vi "LVClass_CorrectionDataManager GetWavefrontCorrectorCurrentPreferences.vi"(0 "CorrectionDataManager in":refnum<class "CorrectionDataManager.lvclass">, 11 "error in (no error)":errorcluster) -> (4 "CorrectionDataManager out":refnum<class "CorrectionDataManager.lvclass">, 8 "Wavefront Corrector State":T1[](array[typedef]), 15 "error out":errorcluster)   [LabVIEW 2020, in "CorrectionDataManager.lvclass"]
doc: "Wavefront corrector actuators preferences getter.\n\n<B>corrdata_managerIn</B> : CorrDataManager object\n<B>corrdata_managerOut</B> : CorrDataManager object\n<B>min</B> : WavefrontCorrector preferences : lowest command value.\n<B>max</B> : WavefrontCorrector preferences : highest command value.\n<B>validity</B> : WavefrontCorrector preferences : status.\n<B>fixed_value</B> : WavefrontCorrector preferences : fixed positions."
uses:
  CorrectionDataManager.lvclass
  Wavefront Corrector states - ONE.ctl
  CorrectionDataManager.lvclass/CorrectionDataManager.ctl
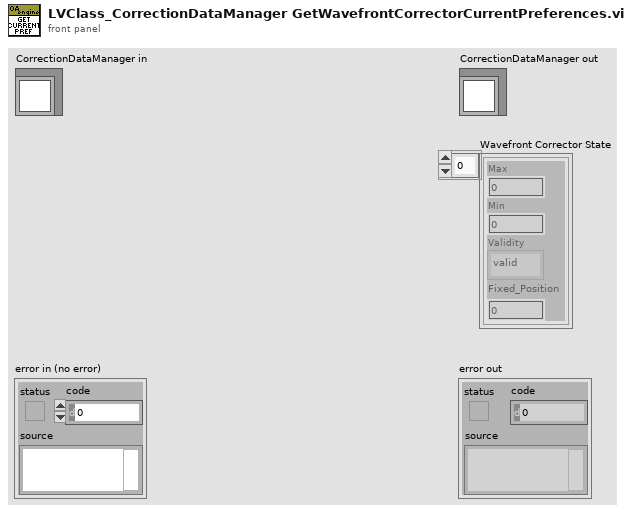
[diagram p1: front panel]
types:
  T1 = typedef "Wavefront Corrector states - ONE.ctl" = cluster{"Max":sgl, "Min":sgl, "Validity":enum16{"valid", "fixed", "invalid"}, "Fixed_Position":sgl}
  T2 = typedef "ClassID.ctl" = i64
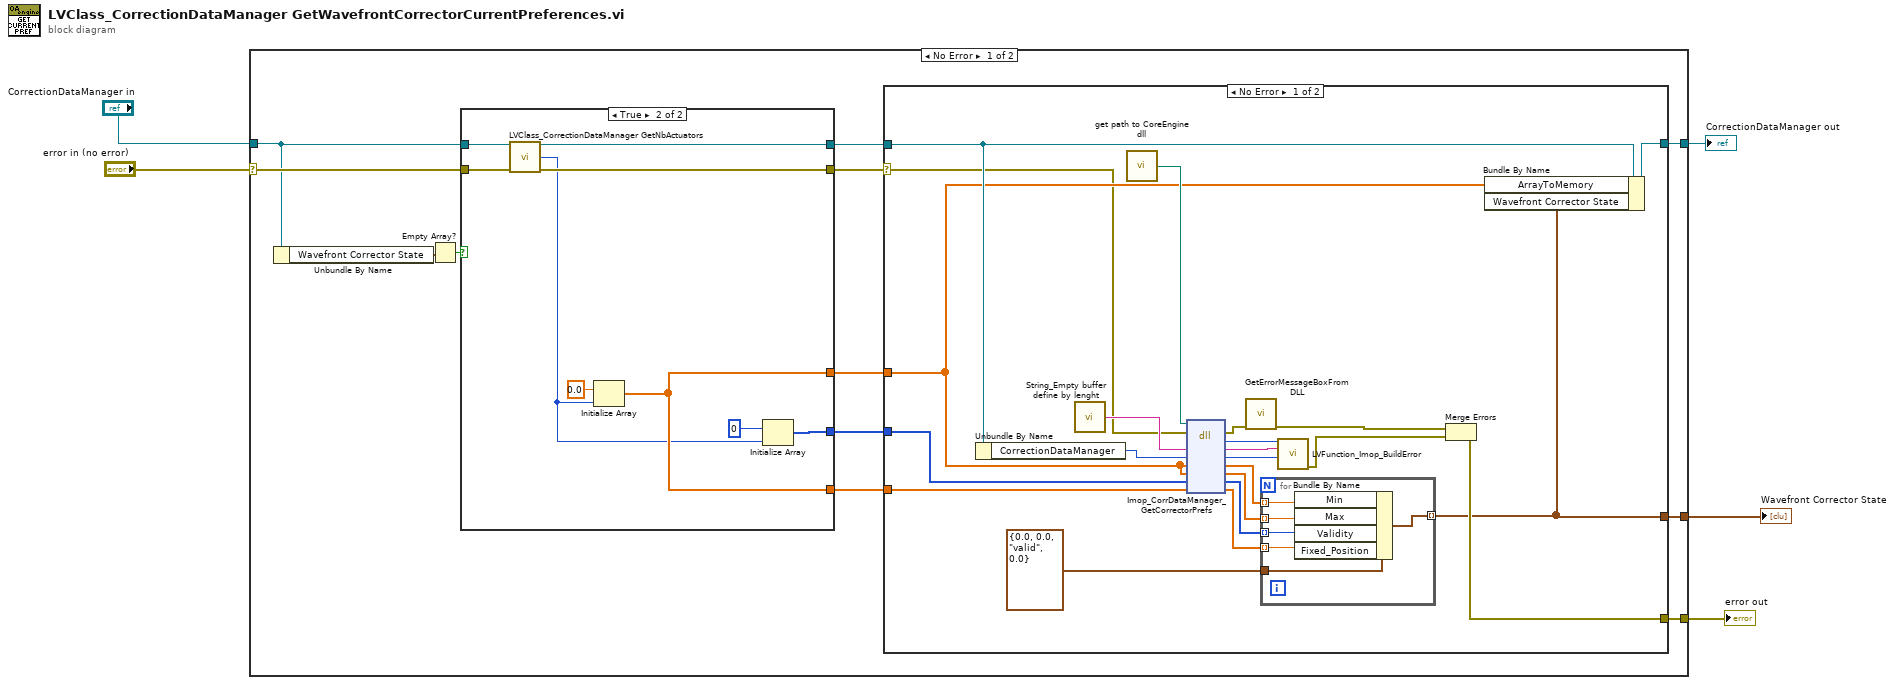
[diagram p0: block diagram]
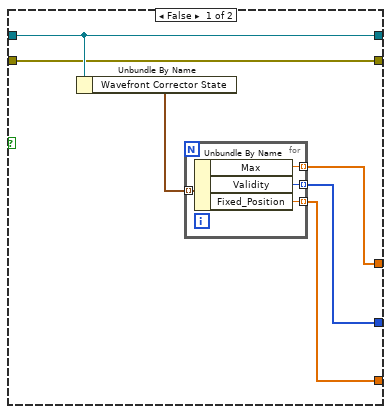
[diagram p3: hidden frame]
diagram:
  n1 = case shown="No Error" "error in (no error)" {
    selector: "error in (no error)" -> [w14 w68]
    tunnel: [w17 w68] -> w4
    tunnel: [w9 w67] -> w5
    tunnel: "CorrectionDataManager in" -> [w13 w67]
    tunnel: [w8 _] -> w1
    frame No Error {
      n2 = Unbundle By Name(w13) -> ("Wavefront Corrector State"=w16:T1[])
      n3 = Empty Array?(array=w16) -> (empty?=w15:bool)
      n4 = case shown="True" w15 {
        tunnel: w13 -> [w53 w64]
        tunnel: [w53 w58] -> w10
        tunnel: [w51 w60] -> w7
        tunnel: [w49 w60] -> w12
        tunnel: w14 -> [w52 w63]
        tunnel: [w52 w62] -> w6
        tunnel: [w50 w61] -> w11
        frame False {
          n5 = Unbundle By Name(w53) -> ("Wavefront Corrector State"=w48:T1[])
          n6 = for {
            tunnel: w48 -> [w57] mode=indexing
            tunnel: [w56] -> w51 mode=indexing
            tunnel: [w55] -> w50 mode=indexing
            tunnel: [w54] -> w49 mode=indexing
            n7 = Unbundle By Name(w57) -> ("Max"=w56:sgl, "Validity"=w55:enum16{"valid", "fixed", "invalid"}, "Fixed_Position"=w54:sgl)
          }
        }
        frame True {
          n8 = call "LVClass_CorrectionDataManager GetNbActuators.vi"("CorrectionDataManager in"=w64, "error in (no error)"=w63) -> ("CorrectionDataManager out"=w58:refnum<class "CorrectionDataManager.lvclass">, "Nb actuators"=w59:i32, "error out"=w62:errorcluster)  [unwired: 11 in]
          n9 = Initialize Array(sgl 0.0, w59) -> (w60:sgl[])
          n10 = Initialize Array(0, w59) -> (w61:i32[])
        }
      }
      n11 = case shown="No Error" w6 {
        selector: w6 -> [w19 w47]
        tunnel: [w32 w47] -> w17
        tunnel: w12 -> [w26 _]
        tunnel: w11 -> [w25 _]
        tunnel: w10 -> [w24 w46]
        tunnel: [w23 w46] -> w9
        tunnel: [w22 _] -> w8
        tunnel: w7 -> [w20 _]
        frame No Error {
          n12 = Unbundle By Name(w24) -> ("CorrectionDataManager"=w31:T2)
          n13 = call "String_Empty buffer define by lenght.vi"() -> ("Empty buffer"=w37:string)  [unwired: 1 in]
          n14 = call "get path to CoreEngine dll.vi"() -> ("path to wavekit library"=w36:path)  [unwired: 14 in, 1 out]
          n15 = dll-call lib="D:/soft/HASO_v3/SVN_trunk/ImOpCoreEngine4_LV2011/DLLs/c_interface_vc100.dll" fn="Imop_CorrDataManager_GetCorrectorPrefs"(path in=w36, error in=w19, "message"=w37, "WavefrontCorrection"=w31, "min"=w20, "max"=w20, "validity"=w25, "fixed_value"=w26) -> (error out=w35:errorcluster, "return type"=w39:i32, "message"=w38:string, "WavefrontCorrection"=w18:i64, "min"=w30:sgl[], "max"=w29:sgl[], "validity"=w28:i32[], "fixed_value"=w27:sgl[])  [unwired: 1 in, 1 out]
          n16 = call "GetErrorMessageBoxFromDLL.vi"("error IN"=w35) -> ("error OUT"=w34:errorcluster)  [unwired: 10 in]
          n17 = for {
            tunnel: w30 -> [w40] mode=indexing
            tunnel: w29 -> [w41] mode=indexing
            tunnel: w28 -> [w45] mode=indexing
            tunnel: w27 -> [w44] mode=indexing
            tunnel: [w43] -> w22 mode=indexing
            tunnel: T1 {"Max"=0.0, "Min"=0.0, "Validity"=enum."valid", "Fixed_Position"=0.0} ("Actuator state") -> [w42]
            n18 = Bundle By Name(cluster=w42, "Min"=w40, "Max"=w41, "Validity"=w45, "Fixed_Position"=w44) -> (w43:T1)
          }
          n19 = call "LVFunction_Imop_BuildError.vi"("code"=w39, "String to Prepend to source (\"\")"=w38, "Adresse"=w18) -> ("error out"=w33:errorcluster)  [unwired: 12 in]
          n20 = Merge Errors(w34, w33) -> (w32:errorcluster)
          n21 = Bundle By Name(cluster=w24, "ArrayToMemory"=w20, "Wavefront Corrector State"=w22) -> (w23:refnum<class "CorrectionDataManager.lvclass">)
        }
        frame Error {
        }
      }
    }
    frame Error {
    }
  }
  "error out" <- w4
  "CorrectionDataManager out" <- w5
  "Wavefront Corrector State" <- w1
